vi "CleanUp.vi"(0 "reference in":refnum<class "ClassReaderNative.lvclass">, 5 "error in (no error)":errorcluster) -> (14 "reference out":refnum<class "ClassReaderNative.lvclass">, 19 "error out":errorcluster)   [LabVIEW 2016, in "ClassReaderNative.lvclass"]
uses:
  <resource>/Framework/Providers/Open_GDS/ClassProviders/Provider_LvNativeClass/ClassReaderNative_class/ClassReaderNative.lvclass
  <resource>/Framework/Providers/Open_GDS/ClassProviders/Provider_LvNativeClass/ClassReaderNative_class/ClassReaderNative.lvclass/ClassReaderNative.ctl
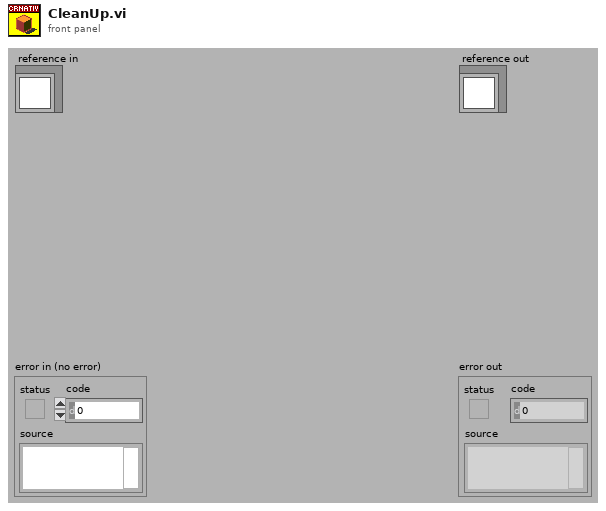
[diagram p1: front panel]
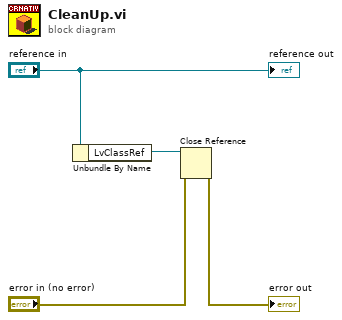
[diagram p0: block diagram]
diagram:
  n1 = Unbundle By Name("reference in") -> ("LvClassRef"=w4:refnum<vi>)
  n2 = Close Reference(reference=w4, error in (no error)="error in (no error)") -> (error out=→"error out":errorcluster)
  "reference out" <- "reference in"
